vi "async process data method.vi"(7 "engine tag data in":T3, 8 "error in":errorcluster, 9 "result transfers in":T1[](array[typedef]), 10 "parameter transfers in":T1[](array[typedef]), 11 "async exec in":T4) -> (0 "error out":errorcluster, 1 "result transfers out":T1[](array[typedef]), 2 "parameter transfers out":T1[](array[typedef]), 3 "async exec out":T4, 5 "engine tag data out":T3)   [LabVIEW 2013, in "main engine.lvlib"]
doc: "Does all the data swapping necessary to map data from an async module to the engine."
uses:
  main engine/main engine.lvlib
  asynchronous executor reference.ctl
  async message to executor.ctl
  Runtime/async command notification.ctl
  <vilib>/NI/Tag Bus/table/data table.ctl
  Runtime/async error info.ctl
  <vilib>/NI/Tag Bus Module Framework/runtime/error classification.ctl
  <vilib>/NI/Tag Bus/table/transfer specification.ctl
  <vilib>/NI/Tag Bus/tag/Data Type.ctl
  <vilib>/NI/Tag Bus/table/data table.lvlib
  <vilib>/NI/Tag Bus/tag/tag descriptor.lvclass
  <vilib>/NI/Tag Bus Module Framework/runtime/TBM module execution interface.lvclass
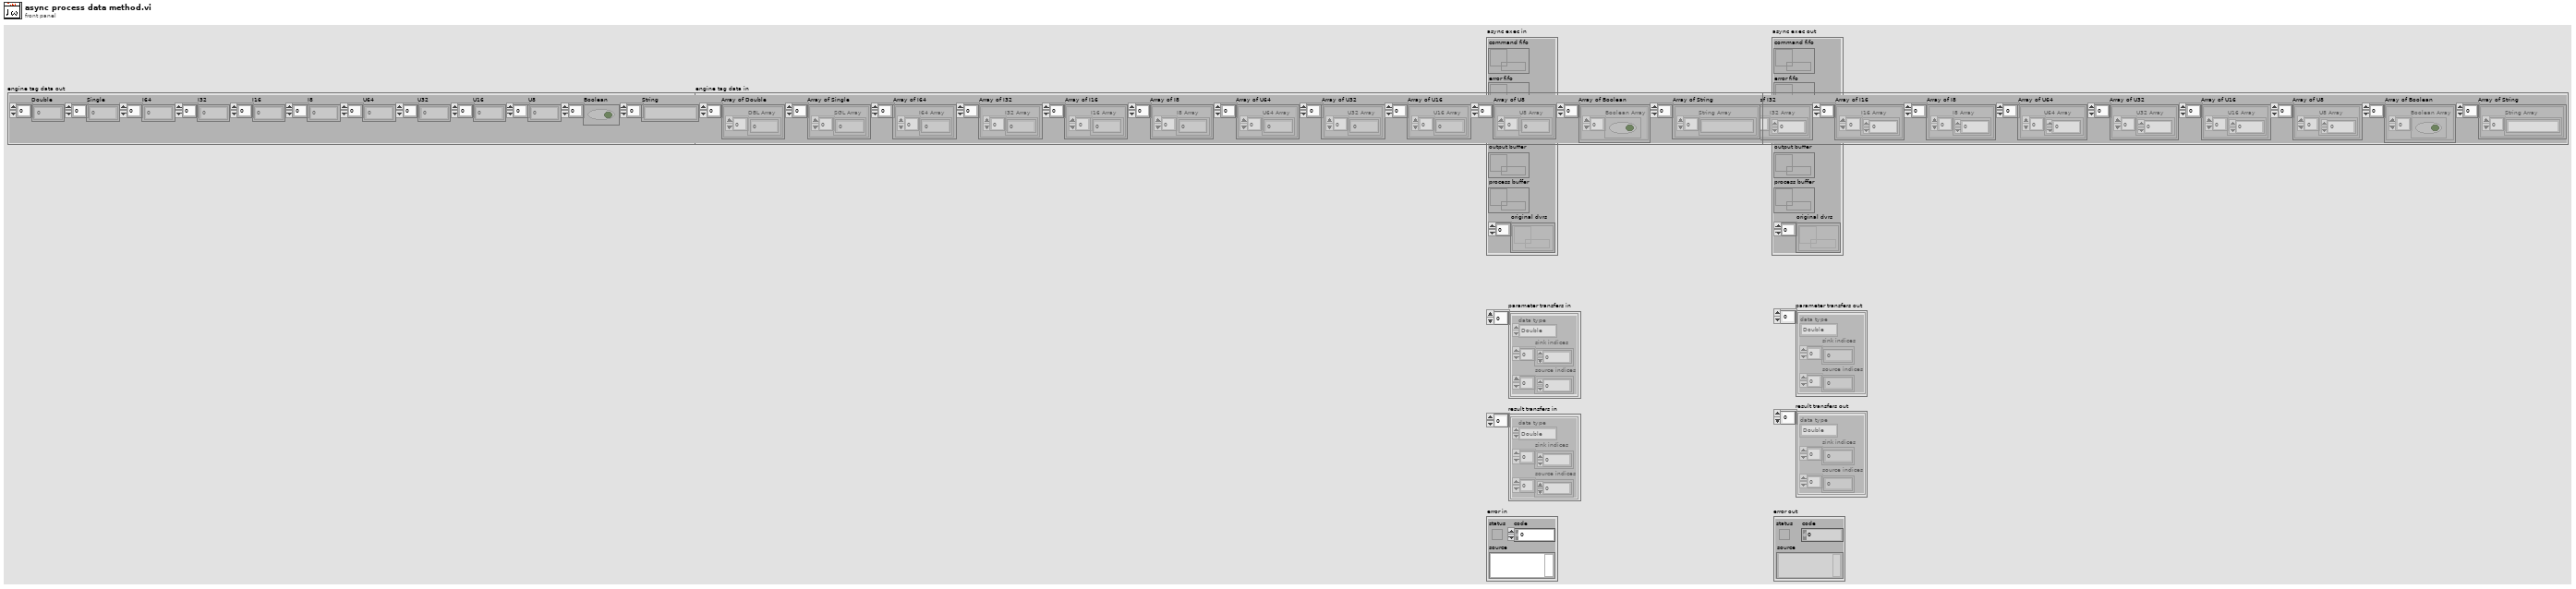
[diagram p1: front panel]
types:
  T1 = typedef "tag bus.lvlib/data table.lvlib/transfer specification.ctl" = cluster{"data type":T2, "sink indices":i32[], "source indices":i32[]}
  T2 = typedef "tag bus.lvlib/tag descriptor.lvclass/Data Type.ctl" = enum16{"Double", "Single", "I64", "I32", "I16", "I8", "U64", "U32", "U16", "U8", "Boolean", "String", "Array of Double", "Array of Single", "Array of I64", "Array of I32", "Array of I16", "Array of I8", "Array of U64", "Array of U32", "Array of U16", "Array of U8", "Array of Boolean", "Array of String"}
  T3 = typedef "tag bus.lvlib/data table.lvlib/data table.ctl" = cluster{"Double":dbl[], "Single":sgl[], "I64":i64[], "I32":i32[], "I16":i16[], "I8":i8[], "U64":u64[], "U32":u32[], "U16":u16[], "U8":u8[], "Boolean":bool[], "String":string[], "Array of Double":cluster{"DBL Array":dbl[]}[], "Array of Single":cluster{"SGL Array":sgl[]}[], "Array of I64":cluster{"I64 Array":i64[]}[], "Array of I32":cluster{"I32 Array":i32[]}[], "Array of I16":cluster{"I16 Array":i16[]}[], "Array of I8":cluster{"I8 Array":i8[]}[], "Array of U64":cluster{"U64 Array":u64[]}[], "Array of U32":cluster{"U32 Array":u32[]}[], "Array of U16":cluster{"U16 Array":u16[]}[], "Array of U8":cluster{"U8 Array":u8[]}[], "Array of Boolean":cluster{"Boolean Array":bool[]}[], "Array of String":cluster{"String Array":string[]}[]}
  T4 = typedef "main engine.lvlib/asynchronous executor reference.ctl" = cluster{"command fifo":refnum<k33>, "error fifo":refnum<k33>, "input buffer":refnum<k33>, "output buffer":refnum<k33>, "process buffer":refnum<k33>, "original dvrs":refnum<data-value>[]}
  T5 = cluster{"parameters":refnum<data-value>, "results":refnum<data-value>}
  T6 = typedef "main engine.lvlib/async command notification.ctl" = enum16{"stop", "input", "process", "output"}
  T7 = typedef "main engine.lvlib/async message to executor.ctl" = cluster{"command":T6, "data 1 (i,o,pp)":refnum<data-value>, "data 2 (pr)":refnum<data-value>, "user value":u64}
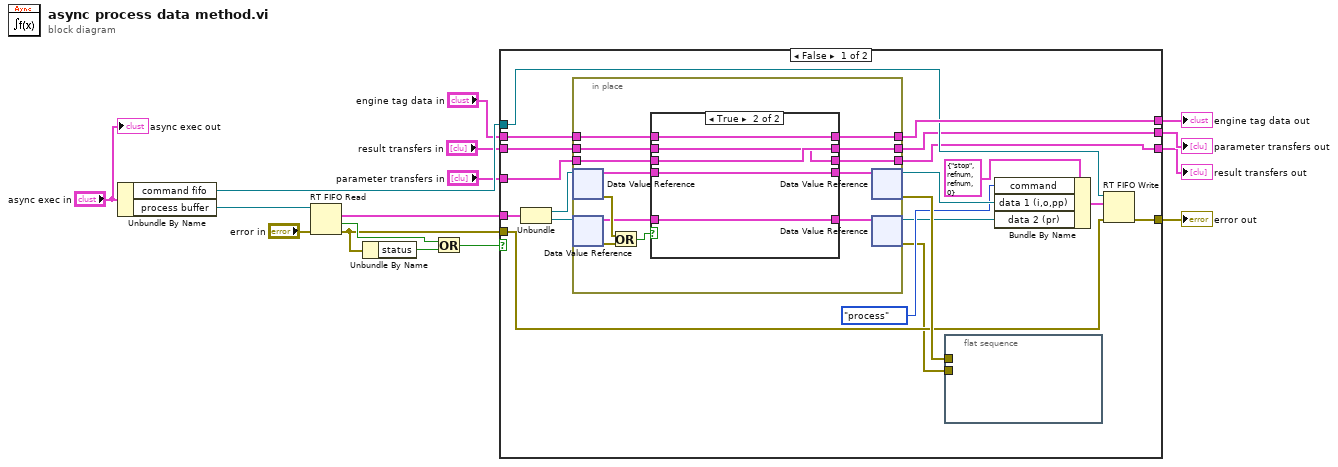
[diagram p0: block diagram]
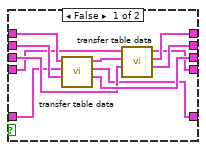
[diagram p2: hidden frame]
diagram:
  n1 = Unbundle By Name("async exec in") -> ("command fifo"=w11:refnum<k33>, "process buffer"=w16:refnum<k33>)
  n2 = RT FIFO Read(0:w16, 3:"error in") -> (9:w15:T5, 10:w14:bool, 11:w12:errorcluster)  [unwired: 2 in, 2 out]
  n3 = Unbundle By Name(w12) -> ("status"=w13:bool)
  n4 = Or(x=w14, y=w13) -> (x .or. y?=w10:bool)
  n5 = case shown="False" w10 {
    tunnel: "engine tag data in" -> [w35 w68]
    tunnel: [w34 w68] -> w8
    tunnel: w15 -> [w32 _]
    tunnel: [w30 w67] -> w9
    tunnel: w12 -> [w31 w67]
    tunnel: w11 -> [w29 _]
    tunnel: [w21 w66] -> w4
    tunnel: "parameter transfers in" -> [w20 w66]
    tunnel: "result transfers in" -> [w18 w65]
    tunnel: [w19 w65] -> w1
    frame False {
      n6 = Unbundle(w32) -> ("parameters"=w24:refnum<data-value>, "results"=w17:refnum<data-value>)
      n7 = in-place {
        in-place-border: w35 -> [w48]
        in-place-border: [w47] -> w34
        in-place-border: [w39] -> w21
        in-place-border: w20 -> [w38]
        in-place-border: [w37] -> w19
        in-place-border: w18 -> [w36]
        n8 = in-place-dvr #1(w24) -> (w45:T3, w46:errorcluster)
        n9 = in-place-dvr #2(w17) -> (w41:T3, w42:errorcluster)
        n10 = Or(x=w46, y=w42) -> (x .or. y?=w43:bool)
        n11 = case shown="True" w43 {
          tunnel: w48 -> [w59 w64]
          tunnel: [w57 w64] -> w47
          tunnel: w45 -> [w52 w63]
          tunnel: [w51 w63] -> w44
          tunnel: w41 -> [w49 w62]
          tunnel: [w50 w62] -> w40
          tunnel: [w54 w61] -> w39
          tunnel: w38 -> [w53 w61]
          tunnel: [w55 w60] -> w37
          tunnel: w36 -> [w56 w60]
          frame False {
            n12 = call <vilib>:"transfer table data.vi"("transfer specification in"=w56, "data table source in"=w49, "data table sink in"=w59) -> ("transfer specification out"=w55:T1[], "data table source out"=w50:T3, "data table sink out"=w58:T3)  [unwired: 6 in]
            n13 = call <vilib>:"transfer table data.vi"("transfer specification in"=w53, "data table source in"=w58, "data table sink in"=w52) -> ("transfer specification out"=w54:T1[], "data table source out"=w57:T3, "data table sink out"=w51:T3)  [unwired: 6 in]
          }
          frame True {
          }
        }
        n14 = in-place-dvr #1(w44) -> (w26:refnum<data-value>, w33:errorcluster)
        n15 = in-place-dvr #2(w40) -> (w23:refnum<data-value>, w22:errorcluster)
      }
      n16 = flat-sequence {
        tunnel: w33 -> [_]
        tunnel: w22 -> [_]
        frame #0 {
        }
      }
      n17 = Bundle By Name(cluster=T7 {"command"=enum."stop", "data 1 (i,o,pp)"=refnum, "data 2 (pr)"=refnum, "user value"=0} ("element"), "command"=async_command_notification."process", "data 1 (i,o,pp)"=w26, "data 2 (pr)"=w23) -> (w27:T7)
      n18 = RT FIFO Write(0:w29, 1:w27, 3:w31) -> (11:w30:errorcluster)  [unwired: 2 in, 3 out]
    }
    frame True {
    }
  }
  "error out" <- w9
  "engine tag data out" <- w8
  "parameter transfers out" <- w4
  "result transfers out" <- w1
  "async exec out" <- "async exec in"
